vi "Sim System Server Set Team.vi"(8 "error in (no error)":errorcluster, 11 "team":string) -> (0 "error out":errorcluster)   [LabVIEW 2026, in "MrcLib.lvlib"]
doc: "Set the team number for a simulated robot."
uses:
  MrcLib.lvlib
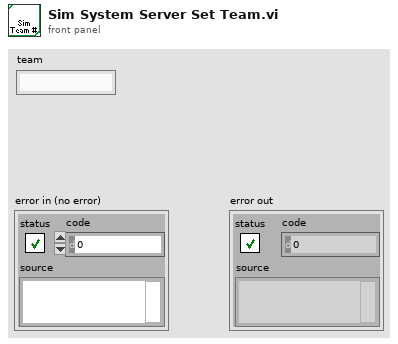
[diagram p1: front panel]
types:
  T1 = typedef "MRC String.ctl" = cluster{"pointer":u64, "length":u64}
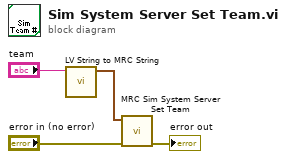
[diagram p0: block diagram]
diagram:
  n1 = call "LV String to MRC String.vi"("LV String"="team") -> ("MRC String"=w1:T1)  [unwired: 10 in]
  n2 = call "MRC Sim System Server Set Team.vi"("error in (no error)"="error in (no error)", "team"=w1) -> ("error out"=→"error out":errorcluster)  [unwired: 9 in]
